vi "1SDI_FPGA_v00.vi"() -> ()   [LabVIEW 2011]
doc: "Controls 6 phase locks based on the interference of two beams at a beam-splitter."
uses:
  Strict Type Defs/Error Signals 1SDI.ctl
  Strict Type Defs/1SDI Lock Point.ctl
  Strict Type Defs/1SDI Output.ctl
  Strict Type Defs/Control 1SDI Input.ctl
  Strict Type Defs/PII individual.ctl
  Strict Type Defs/Error Scale 1SDI.ctl
  Strict Type Defs/Lock Thresh 1SDI.ctl
  Strict Type Defs/Theta graph.ctl
  Strict Type Defs/Safety First.ctl
  Strict Type Defs/Scope.ctl
  Strict Type Defs/1SDI Max.ctl
  Strict Type Defs/1SDI Min.ctl
  <vilib>/rvi/interface/RandomDataEmulation/nirviRandomDataFPGAFIFO.vi
  <vilib>/rvi/interface/RandomDataEmulation/niFpgaRandomDataHandleErrors.vi
  <vilib>/rvi/DataTransferAndStorage/Container/XNode/niFpgaContainer.xnode
  <vilib>/rvi/interface/RandomDataEmulation/nirviRandomDataFpgaReadWriteTemplate.vi
panel:
  out "Min":T1
  out "Max":T2
  in  "Graph Delay(uSec)":u32 caption="Count(uSec)"
  out "HD Errors xp":T3
  in  "Scope":T4={"Trigger Direction"=enum."plus-minus", "Delay"=0, "Aquisition Rate (Ticks)"=40, "Offset"=0, "Channel"=0, "Channel Selector"={"Channel 1"=0, "Channel 2"=4, "Channel 3"=8, "Channel 4"=8}} {"Channel Selector"."Channel 4" items=["Error Signal 1", "Error Signal 2", "Scan Trigger 1", "Scan Trigger 2", "DC Signal 1", "DC Signal 2", "PI Out 1", "PI Out 2"]; "Channel Selector"."Channel 3" items=["Error Signal 1", "Error Signal 2", "Scan Trigger 1", "Scan Trigger 2", "DC Signal 1", "DC Signal 2", "PI Out 1", "PI Out 2"]; "Channel Selector"."Channel 2" items=["Error Signal 1", "Error Signal 2", "Scan Trigger 1", "Scan Trigger 2", "DC Signal 1", "DC Signal 2", "PI Out 1", "PI Out 2"]; "Channel Selector"."Channel 1" items=["Error Signal 1", "Error Signal 2", "Scan Trigger 1", "Scan Trigger 2", "DC Signal 1", "DC Signal 2", "PI Out 1", "PI Out 2"]}
  in  "quit Control Loop":bool
  in  "Control":T5={"PII In 1"={"Lock"=FALSE, "Hold"=FALSE, "P Gain"=0, "P BS"=-5, "I Gain"=0, "I BS"=-10, "I2 G"=0, "I2 BS"=-26, "Scan Amp"=0, "Scan Off"=0, "Scan FS"=0, "SFS BS"=0, "I Max value"=10000, "I2 Max value"=10000, "Scope.Offset"=0, "Trigger Direction"=enum."either", "Scan-PII thresh"=0}, "PII In 2"={"Lock"=FALSE, "Hold"=FALSE, "P Gain"=0, "P BS"=-10, "I Gain"=0, "I BS"=-10, "I2 G"=0, "I2 BS"=-26, "Scan Amp"=0, "Scan Off"=0, "Scan FS"=0, "SFS BS"=0, "I Max value"=10000, "I2 Max value"=10000, "Scope.Offset"=0, "Trigger Direction"=enum."either", "Scan-PII thresh"=0}, "PII In 3"={"Lock"=FALSE, "Hold"=FALSE, "P Gain"=0, "P BS"=-10, "I Gain"=0, "I BS"=-10, "I2 G"=0, "I2 BS"=-26, "Scan Amp"=0, "Scan Off"=0, "Scan FS"=0, "SFS BS"=0, "I Max value"=10000, "I2 Max value"=10000, "Scope.Offset"=0, "Trigger Direction"=enum."either", "Scan-PII thresh"=0}, "Error scale"={"Pre-Offset"={"Pre-Offset 1"=2, "Pre-Offset 2"=0, "Pre-Offset 3"=0, "Pre-Offset 4"=0, "Pre-Offset 5"=2}, "Post-Offset "={"Offset 1"=0, "Offset 2"=300, "Offset 3"=0, "Offset 4"=0, "Offset 5"=0}, "Gains"={"Gain 1"=0, "Gain 2"=300, "Gain 3"=0, "Gain 4"=0, "Gain 5"=0}, "Bit Shifts"={"Bit Shift 1"=0, "Bit Shift 2"=300, "Bit Shift 3"=0, "Bit Shift 4"=0, "Bit Shift 5"=0}}, "Lock Thresh"={"EPR"=2, "HD A"=0, "HD B"=10}, "Re-Scan Thresh"={"EPR"=2, "HD A"=0, "HD B"=0}, "Theta"={"HD A Sin Theta"=0, "HD A Cos Theta"=0, "HD B Sin Theta"=0, "HD B Cos Theta"=0}, "Safety First"={"lim reset"=FALSE, "no limit"=FALSE, "pos slew rate * dt"=0, "neg slew rate * dt"=-10, "Hold All"=FALSE, "Count(Ticks)"=0}}
  in  "\"I too high?\"":T11
  in  "\"Outputs\"":T12
  out "Outputs":T12={"EPR"=-270, "HD A"=-1710, "HD B"=880}
  in  "\"Trigger\"":T11
  out "Trigger":T11
  out "Cavity Errors":T13={"EPR"=0, "HD A"=1800, "HD B"=0}
  out "Control Loop count":i32=11285327
  out "Scope Full?":bool
  out "Scope loop count":i32=119818
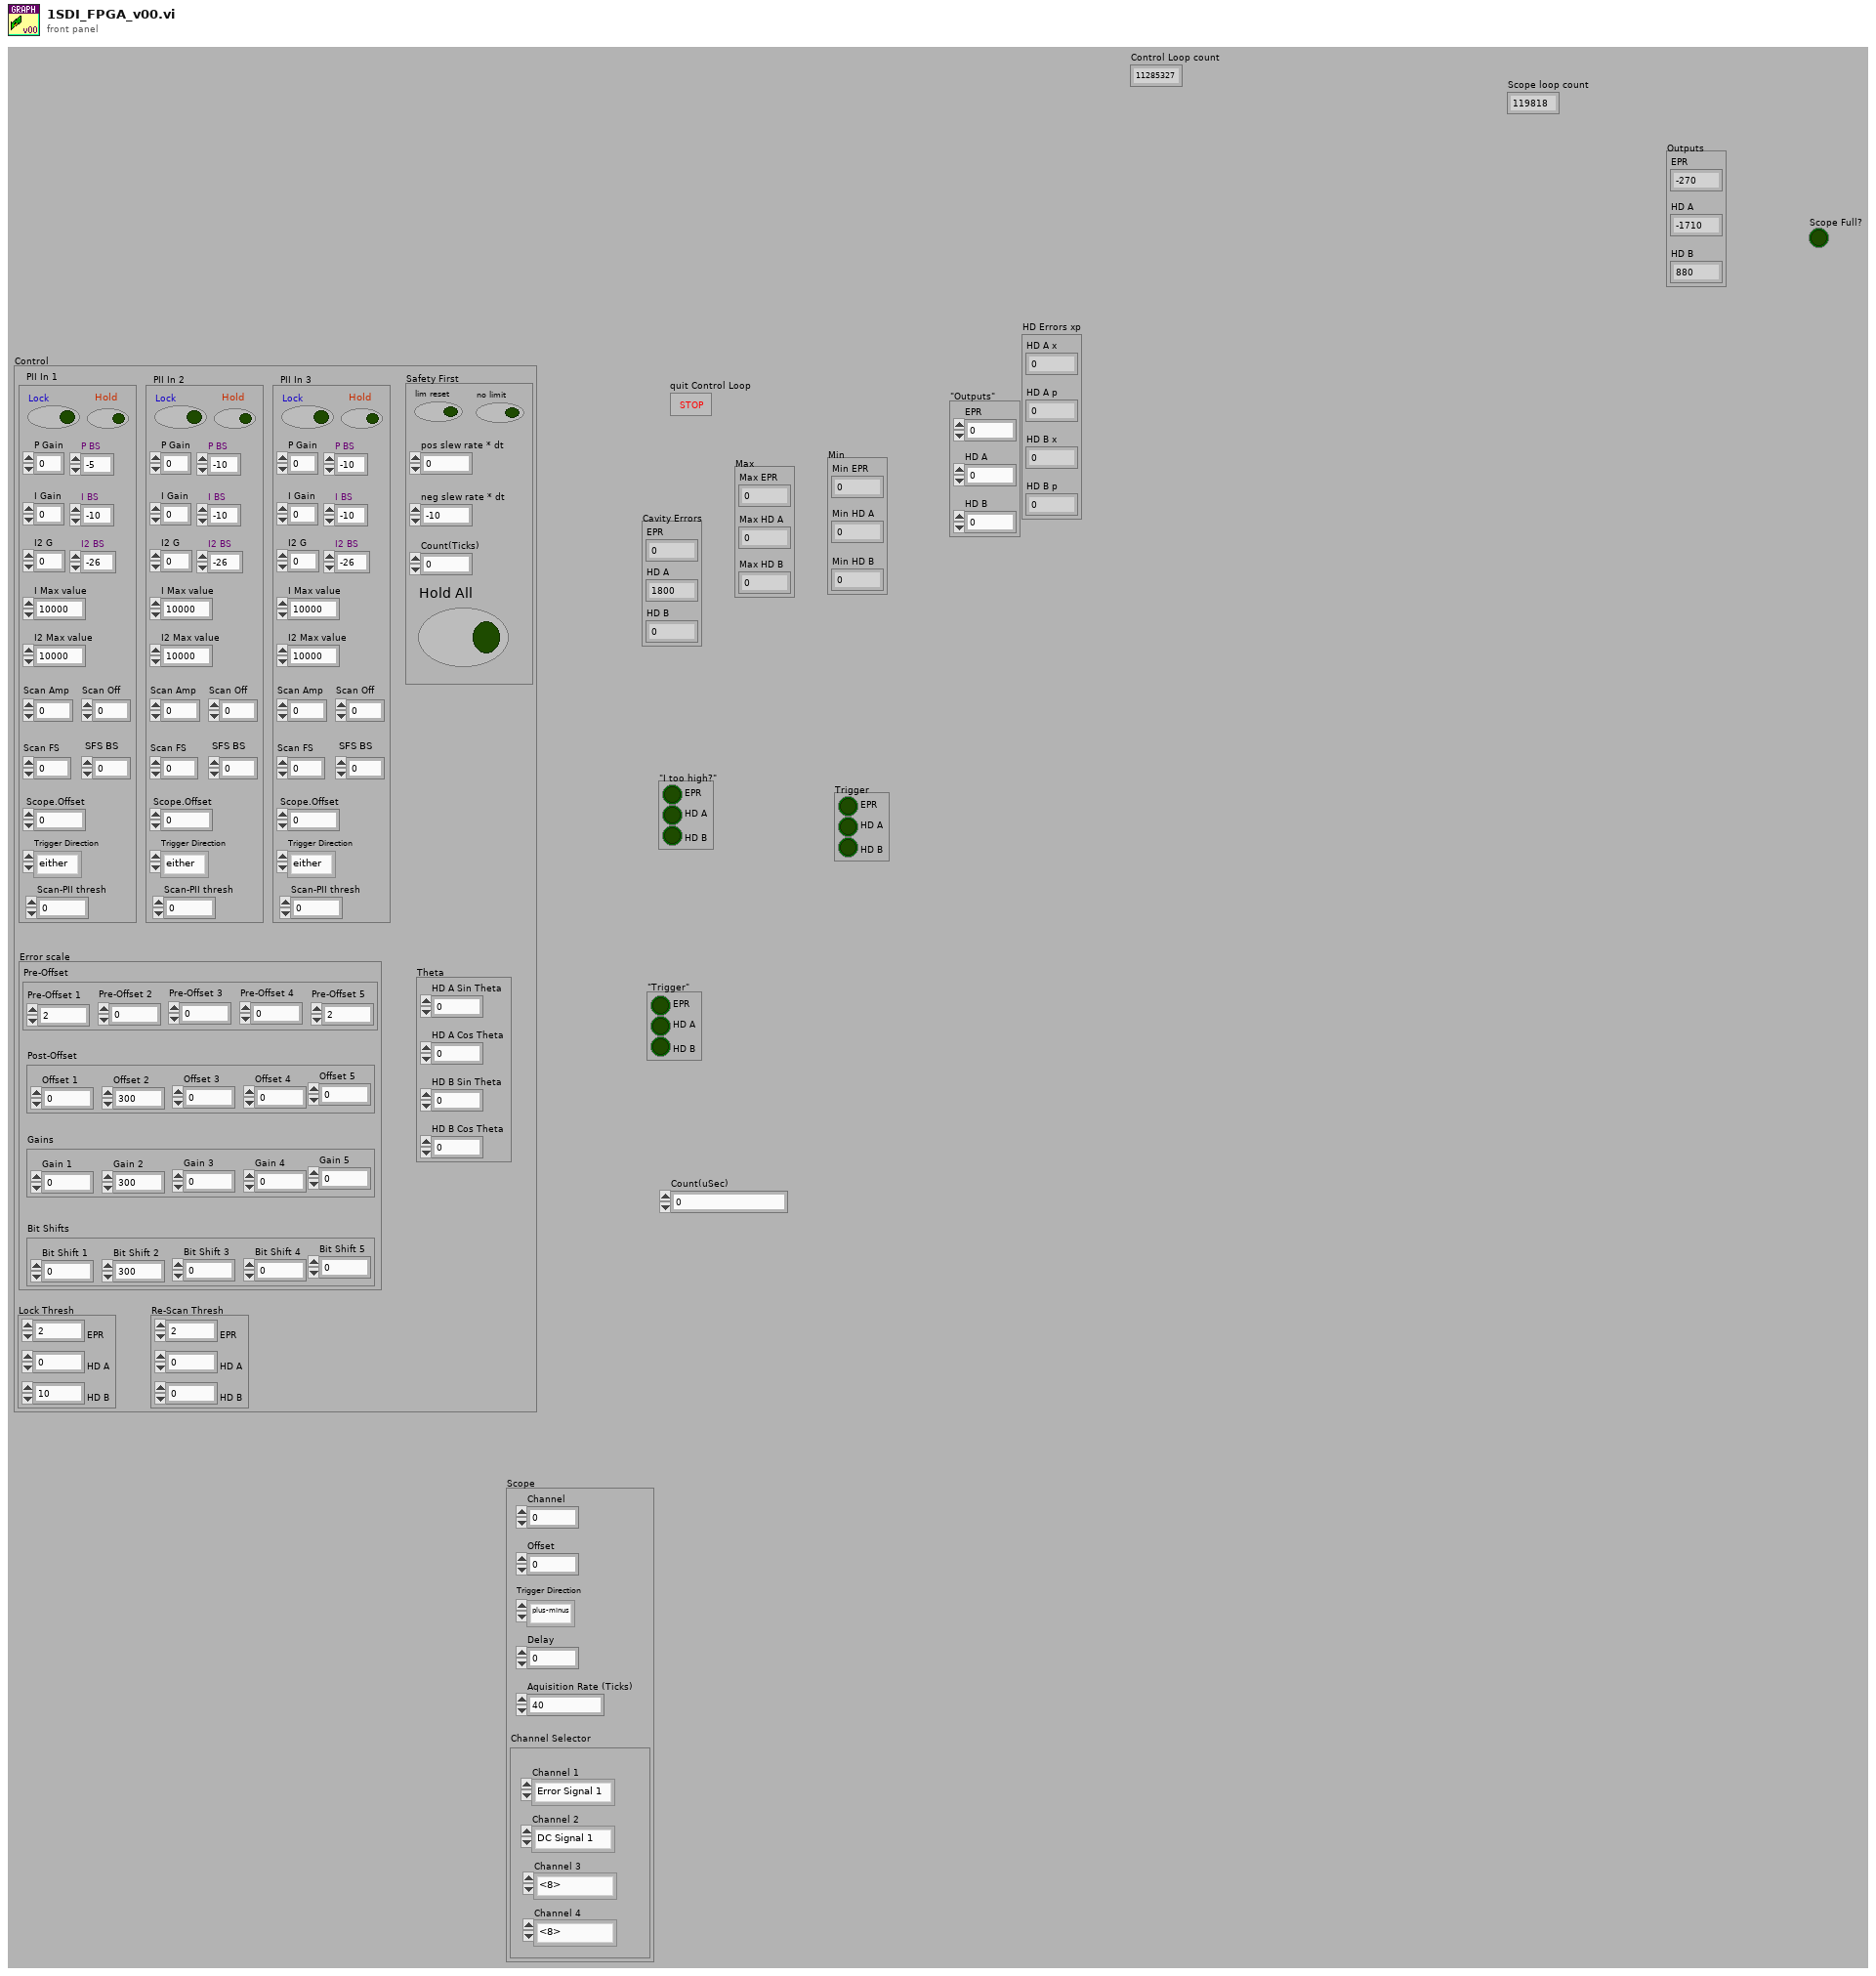
[diagram p1: front panel]
types:
  T1 = typedef "1SDI Min.ctl" = cluster{"Min EPR":i16, "Min HD A":i16, "Min HD B":i16}
  T2 = typedef "1SDI Max.ctl" = cluster{"Max EPR":i16, "Max HD A":i16, "Max HD B":i16}
  T3 = cluster{"HD A x":i16, "HD A p":i16, "HD B x":i16, "HD B p":i16}
  T4 = typedef "Scope.ctl" = cluster{"Trigger Direction":enum8{"either", "minus-plus", "plus-minus"}, "Delay":u32, "Aquisition Rate (Ticks)":u32, "Offset":i16, "Channel":i32, "Channel Selector":cluster{"Channel 1":i32, "Channel 2":i32, "Channel 3":i32, "Channel 4":i32}}
  T5 = typedef "Control 1SDI Input.ctl" = cluster{"PII In 1":T6, "PII In 2":T6, "PII In 3":T6, "Error scale":T7, "Lock Thresh":T8, "Re-Scan Thresh":T8, "Theta":T9, "Safety First":T10}
  T6 = typedef "PII individual.ctl" = cluster{"Lock":bool, "Hold":bool, "P Gain":i32, "P BS":i16, "I Gain":i32, "I BS":i16, "I2 G":i32, "I2 BS":i16, "Scan Amp":i16, "Scan Off":i16, "Scan FS":u16, "SFS BS":i16, "I Max value":i32, "I2 Max value":i32, "Scope.Offset":i16, "Trigger Direction":enum8{"either", "minus-plus", "plus-minus"}, "Scan-PII thresh":i16}
  T7 = typedef "Error Scale 1SDI.ctl" = cluster{"Pre-Offset":cluster{"Pre-Offset 1":i16, "Pre-Offset 2":i16, "Pre-Offset 3":i16, "Pre-Offset 4":i16, "Pre-Offset 5":i16}, "Post-Offset ":cluster{"Offset 1":i16, "Offset 2":i16, "Offset 3":i16, "Offset 4":i16, "Offset 5":i16}, "Gains":cluster{"Gain 1":i16, "Gain 2":i16, "Gain 3":i16, "Gain 4":i16, "Gain 5":i16}, "Bit Shifts":cluster{"Bit Shift 1":i16, "Bit Shift 2":i16, "Bit Shift 3":i16, "Bit Shift 4":i16, "Bit Shift 5":i16}}
  T8 = typedef "Lock Thresh 1SDI.ctl" = cluster{"EPR":i16, "HD A":i16, "HD B":i16}
  T9 = typedef "Theta graph.ctl" = cluster{"HD A Sin Theta":i32, "HD A Cos Theta":i32, "HD B Sin Theta":i32, "HD B Cos Theta":i32}
  T10 = typedef "Safety First.ctl" = cluster{"lim reset":bool, "no limit":bool, "pos slew rate * dt":i16, "neg slew rate * dt":i16, "Hold All":bool, "Count(Ticks)":u32}
  T11 = typedef "1SDI Lock Point.ctl" = cluster{"EPR":bool, "HD A":bool, "HD B":bool}
  T12 = typedef "1SDI Output.ctl" = cluster{"EPR":i16, "HD A":i16, "HD B":i16}
  T13 = typedef "Error Signals 1SDI.ctl" = cluster{"EPR":i16, "HD A":i16, "HD B":i16}
  T14 = typedef "Signals 1SDI.ctl" = cluster{"PII In 1":T6, "PII In 2":T6, "PII In 3":T6, "Lock Thresh":T8, "Re-Scan Thresh":T8, "Safety First":T10, "Graph Errors":T13}
  T15 = typedef "1SDI Control Cluster.ctl" = cluster{"Control EPR":T6, "Control HD A":T6, "Control HD B":T6, "Max":T2, "Min":T1, "Lock Threshold":T8, "Re-Scan Threshold":T8, "Lock Point?":T11, "Re-scan?":T11, "Lock pressed? (-1)":T11, "Cavity Errors":T13, "State (-1)":T16, "Safety First":T10}
  T16 = typedef "1SDI State.ctl" = cluster{"EPR":enum16{"Safe", "Hold", "Scan", "Lock"}, "HD A":enum16{"Safe", "Hold", "Scan", "Lock"}, "HD B":enum16{"Safe", "Hold", "Scan", "Lock"}}
  T17 = typedef "1SDI PII Scan State.ctl" = cluster{"Control EPR":T6, "Control HD A":T6, "Control HD B":T6, "Error Signals":T13, "State":T16}
  T18 = typedef "1SDI MaxMin.ctl" = cluster{"State":T16, "Reset MaxMin?":T19, "Max":T2, "Min":T1, "Lock pressed?":T11, "Safety First":T10}
  T19 = typedef "1SDI Reset MaxMin.ctl" = cluster{"EPR":bool, "HD A":bool, "HD B":bool}
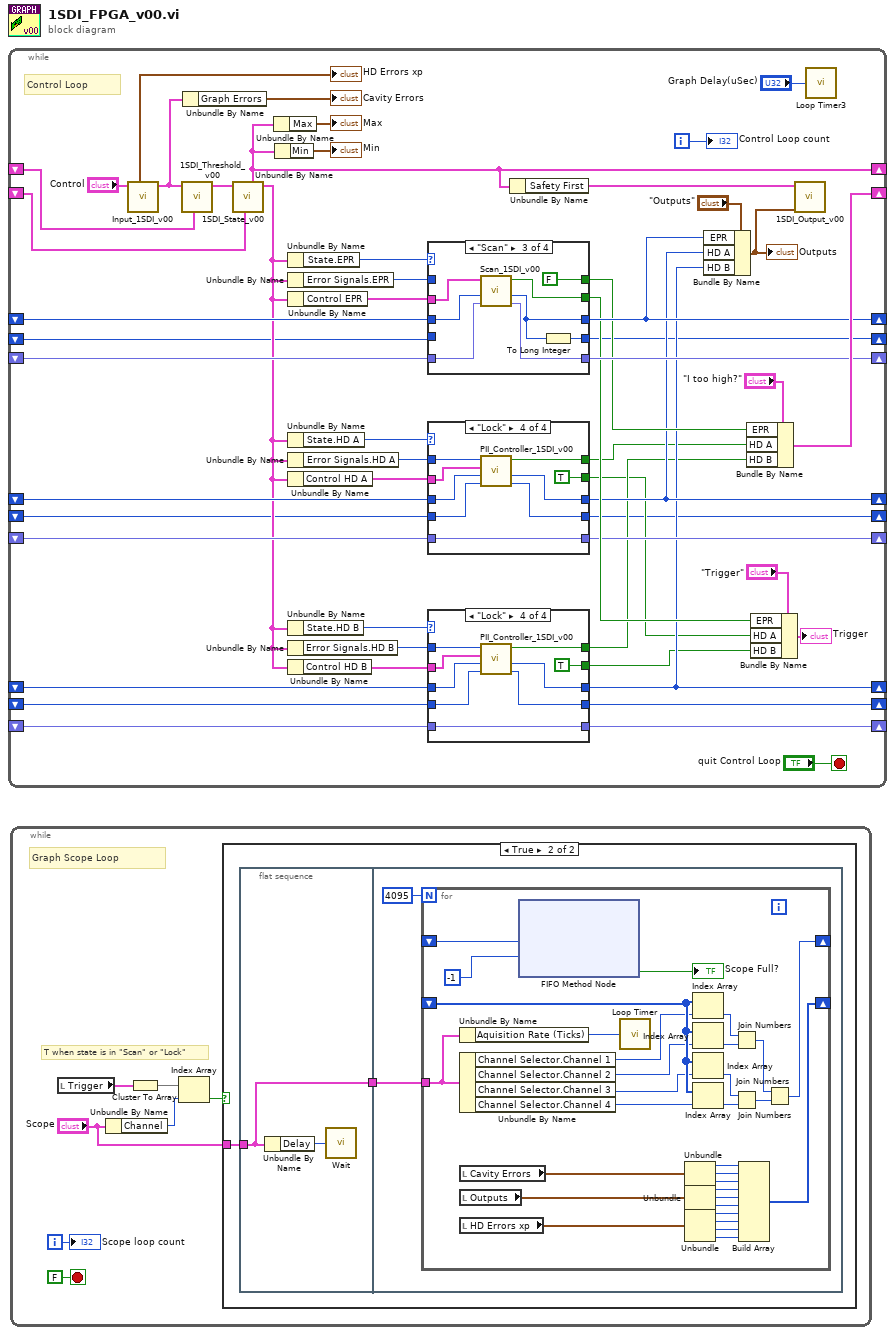
[diagram p0: block diagram]
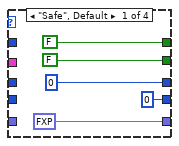
[diagram p3: hidden frame]
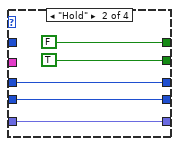
[diagram p4: hidden frame]
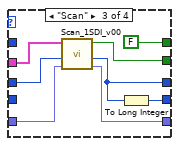
[diagram p5: hidden frame]
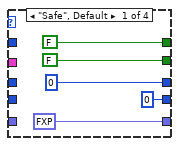
[diagram p6: hidden frame]
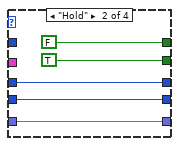
[diagram p7: hidden frame]
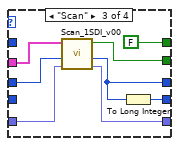
[diagram p8: hidden frame]
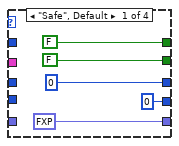
[diagram p9: hidden frame]
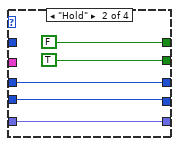
[diagram p10: hidden frame]
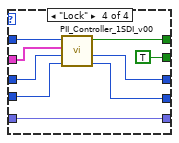
[diagram p11: hidden frame]
diagram:
  n1 = while {
    shift-right: [w53] -> _
    shift-left: _ -> [w48]
    shift-right: [w19] -> _
    shift-left: _ -> [w47]
    shift-right: [w41] -> _
    shift-left: _ -> [w46]
    shift-right: [w45] -> _
    shift-left: _ -> [w44]
    shift-right: [w30] -> _
    shift-left: _ -> [w36]
    shift-right: [w35] -> _
    shift-left: _ -> [w34]
    shift-right: [w2] -> _
    shift-left: _ -> [w1]
    shift-right: [w29] -> _
    shift-left: _ -> [w31]
    shift-right: [w32] -> _
    shift-left: _ -> [w33]
    shift-right: [w6] -> _
    shift-left: _ -> [w5]
    shift-right: [w4] -> _
    shift-left: _ -> [w3]
    i -> [w49]
    stop <- "quit Control Loop" stop-if-true
    # "Control Loop"
    n2 = call "Input_1SDI_v00.vi"("Control"="Control") -> ("Signals"=w24:T14, "HD Errors xp"=→"HD Errors xp":T3)  [unwired: 9 in]
    n3 = call "1SDI_Threshold_v00.vi"("MaxMin"=w47, "Signals"=w24) -> ("Control Graph Cluster"=w21:T15)  [unwired: 9 in]
    n4 = Unbundle By Name(w24) -> ("Graph Errors"=→"Cavity Errors":T13)
    n5 = call "1SDI_State_v00.vi"("\"I too high?\""=w48, "Control Cavity Cluster"=w21) -> ("PII Scan State Errors"=w8:T17, "MaxMin"=w19:T18)  [unwired: 8 in]
    n6 = Unbundle By Name(w19) -> ("Max"=→"Max":T2)
    n7 = Unbundle By Name(w19) -> ("Min"=→"Min":T1)
    n8 = Unbundle By Name(w8) -> ("State.EPR"=w15:enum16{"Safe", "Hold", "Scan", "Lock"})
    n9 = Unbundle By Name(w8) -> ("Error Signals.EPR"=w16:i16)
    n10 = Unbundle By Name(w8) -> ("Control EPR"=w17:T6)
    n11 = Unbundle By Name(w8) -> ("State.HD A"=w14:enum16{"Safe", "Hold", "Scan", "Lock"})
    n12 = Unbundle By Name(w8) -> ("Error Signals.HD A"=w13:i16)
    n13 = Unbundle By Name(w8) -> ("Control HD A"=w12:T6)
    n14 = Unbundle By Name(w8) -> ("State.HD B"=w9:enum16{"Safe", "Hold", "Scan", "Lock"})
    n15 = Unbundle By Name(w8) -> ("Error Signals.HD B"=w11:i16)
    n16 = Unbundle By Name(w8) -> ("Control HD B"=w10:T6)
    n17 = case shown="\"Scan\"" w15 {
      tunnel: w16 -> [_ _ _ w135]
      tunnel: [FALSE ("I too high? (F=No)") FALSE ("I too high? (F=No)") FALSE ("I too high? (F=No)") w134] -> w40
      tunnel: w17 -> [_ _ w125 w133]
      tunnel: [i16 0 ("PII out") w117 w119 w130] -> w41
      tunnel: w46 -> [_ w117 w122 w131]
      tunnel: w3 -> [_ w114 _ w127]
      tunnel: [fxp<+,33,17> 0.0 ("Scan") w116 w124 w129] -> w45
      tunnel: w44 -> [_ w116 w123 w129]
      tunnel: [FALSE ("Zero Crossing") TRUE ("Zero Crossing") w121 TRUE ("Zero Crossing")] -> w39
      tunnel: [0 ("I Cavity") w114 w120 w128] -> w4
      frame "Safe", Default {
      }
      frame "Hold" {
      }
      frame "Scan" {
        n18 = call "Scan_1SDI_v00.vi"("Scan (-1)"=w123, "Scan out (-1)"=w122, "Control Cavity"=w125) -> ("Scan"=w124:fxp<+,33,17>, "Scan out"=w119:i16, "Zero Crossing"=w121:bool)  [unwired: 6 in]
        n19 = To Long Integer(number=w119) -> (32bit integer=w120:i32)
      }
      frame "Lock" {
        n20 = call "PII_Controller_1SDI_v00.vi"("Integrator (-1)"=w127, "PII out (-1)"=w131, "Control Cavity"=w133, "OPO A Error"=w135) -> ("I Cavity"=w128:i32, "PII out"=w130:i16, "I too high?"=w134:bool)  [unwired: 5 in]
      }
    }
    n21 = case shown="\"Lock\"" w14 {
      tunnel: w13 -> [_ _ _ w108]
      tunnel: [FALSE ("I too high? (F=No)") FALSE ("I too high? (F=No)") FALSE ("I too high? (F=No)") w107] -> w28
      tunnel: w12 -> [_ _ w98 w105]
      tunnel: [i16 0 ("PII out") w90 w92 w102] -> w30
      tunnel: w36 -> [_ w90 w95 w103]
      tunnel: w5 -> [_ w87 _ w106]
      tunnel: [fxp<+,33,17> 0.0 ("Scan") w89 w97 w101] -> w35
      tunnel: w34 -> [_ w89 w96 w101]
      tunnel: [FALSE ("Zero Crossing") TRUE ("Zero Crossing") w94 TRUE ("Zero Crossing")] -> w26
      tunnel: [0 ("I Cavity") w87 w93 w100] -> w6
      frame "Safe", Default {
      }
      frame "Hold" {
      }
      frame "Scan" {
        n22 = call "Scan_1SDI_v00.vi"("Scan (-1)"=w96, "Scan out (-1)"=w95, "Control Cavity"=w98) -> ("Scan"=w97:fxp<+,33,17>, "Scan out"=w92:i16, "Zero Crossing"=w94:bool)  [unwired: 6 in]
        n23 = To Long Integer(number=w92) -> (32bit integer=w93:i32)
      }
      frame "Lock" {
        n24 = call "PII_Controller_1SDI_v00.vi"("Integrator (-1)"=w106, "PII out (-1)"=w103, "Control Cavity"=w105, "OPO A Error"=w108) -> ("I Cavity"=w100:i32, "PII out"=w102:i16, "I too high?"=w107:bool)  [unwired: 5 in]
      }
    }
    n25 = case shown="\"Lock\"" w9 {
      tunnel: w11 -> [_ _ _ w81]
      tunnel: [FALSE ("I too high? (F=No)") FALSE ("I too high? (F=No)") FALSE ("I too high? (F=No)") w80] -> w27
      tunnel: w10 -> [_ _ w71 w79]
      tunnel: [i16 0 ("PII out") w63 w66 w76] -> w29
      tunnel: w31 -> [_ w63 w68 w77]
      tunnel: [fxp<+,33,17> 0.0 ("Scan") w62 w70 w75] -> w32
      tunnel: w33 -> [_ w62 w69 w75]
      tunnel: [FALSE ("Zero Crossing") TRUE ("Zero Crossing") w67 TRUE ("Zero Crossing")] -> w25
      tunnel: [0 ("I Cavity") w60 w65 w74] -> w2
      tunnel: w1 -> [_ w60 _ w73]
      frame "Safe", Default {
      }
      frame "Hold" {
      }
      frame "Scan" {
        n26 = call "Scan_1SDI_v00.vi"("Scan (-1)"=w69, "Scan out (-1)"=w68, "Control Cavity"=w71) -> ("Scan"=w70:fxp<+,33,17>, "Scan out"=w66:i16, "Zero Crossing"=w67:bool)  [unwired: 6 in]
        n27 = To Long Integer(number=w66) -> (32bit integer=w65:i32)
      }
      frame "Lock" {
        n28 = call "PII_Controller_1SDI_v00.vi"("Integrator (-1)"=w73, "PII out (-1)"=w77, "Control Cavity"=w79, "OPO A Error"=w81) -> ("I Cavity"=w74:i32, "PII out"=w76:i16, "I too high?"=w80:bool)  [unwired: 5 in]
      }
    }
    n29 = Unbundle By Name(w19) -> ("Safety First"=w43:T10)
    n30 = Bundle By Name(cluster="\"Outputs\"", "EPR"=w41, "HD A"=w30, "HD B"=w29) -> (w42:T12)
    "Outputs" <- w42
    n31 = Bundle By Name(cluster="\"I too high?\"", "EPR"=w40, "HD A"=w28, "HD B"=w27) -> (w53:T11)
    n32 = Bundle By Name(cluster="\"Trigger\"", "EPR"=w39, "HD A"=w26, "HD B"=w25) -> (→"Trigger":T11)
    n33 = call "1SDI_Output_v00.vi"("Outputs"=w42, "Safety First"=w43) -> ()  [unwired: 10 in]
    n34 = call "Loop Timer3"("Count(uSec)"="Graph Delay(uSec)") -> ()  [unwired: 1 out]
    "Control Loop count" <- w49
  }
  n35 = while {
    i -> [w139]
    stop <- FALSE ("stop") stop-if-true
    # "Graph Scope Loop"
    # "T when state is in \"Scan\" or \"Lock\""
    n36 = local read "Trigger"() -> (w137:T11)
    n37 = Unbundle By Name("Scope") -> ("Channel"=w140:i32)
    n38 = Cluster To Array(cluster=w137) -> (array=w141:bool[])
    n39 = Index Array(array=w141, index=w140) -> (element=w138:bool)
    n40 = case shown="True" w138 {
      tunnel: "Scope" -> [_ w144]
      frame False {
      }
      frame True {
        n41 = flat-sequence {
          tunnel: w144 -> [w145]
          tunnel: [w145] -> w143
          tunnel: w143 -> [w147]
          frame #0 {
            n42 = Unbundle By Name(w145) -> ("Delay"=w146:u32)
            n43 = call "Wait"("Count(Ticks)"=w146) -> ()  [unwired: 1 out]
          }
          frame #1 {
            n44 = for {
              N: 4095 -> [_]
              tunnel: w147 -> [w178]
              shift-right: [w170] -> _
              shift-left: _ -> [w169]
              shift-right: [w165] -> _
              shift-left: _ -> [w164]
              n45 = Unbundle By Name(w178) -> ("Aquisition Rate (Ticks)"=w179:u32)
              n46 = Unbundle By Name(w178) -> ("Channel Selector.Channel 1"=w166:i32, "Channel Selector.Channel 2"=w167:i32, "Channel Selector.Channel 3"=w161:i32, "Channel Selector.Channel 4"=w168:i32)
              n47 = local read "Cavity Errors"() -> (w177:T13)
              n48 = local read "Outputs"() -> (w176:T12)
              n49 = local read "HD Errors xp"() -> (w159:T3)
              n50 = xnode ("FIFO Method Node")("Element"=w164, "Timeout"=-1) -> ("Timed Out?"=→"Scope Full?":bool)  [unwired: 1 in, 1 out]
              n51 = call "Loop Timer"("Count(uSec)"=w179) -> ()  [unwired: 1 out]
              n52 = Unbundle(w177) -> ("EPR"=w149:i16, "HD A"=w150:i16, "HD B"=w151:i16)
              n53 = Unbundle(w176) -> ("EPR"=w152:i16, "HD A"=w153:i16, "HD B"=w154:i16)
              n54 = Unbundle(w159) -> ("HD A x"=w158:i16, "HD A p"=w157:i16, "HD B x"=w156:i16, "HD B p"=w155:i16)
              n55 = Index Array(array=w169, index=w166) -> (element=w172:i16)
              n56 = Index Array(array=w169, index=w167) -> (element=w171:i16)
              n57 = Index Array(array=w169, index=w161) -> (element=w160:i16)
              n58 = Index Array(array=w169, index=w168) -> (element=w173:i16)
              n59 = Join Numbers(hi=w172, lo=w171) -> ((hi.lo)=w175:u32)
              n60 = Join Numbers(hi=w160, lo=w173) -> ((hi.lo)=w174:u32)
              n61 = Build Array(w149, w150, w151, w152, w153, w154, w158, w157, w156, w155) -> (w170:i16[])
              n62 = Join Numbers(hi=w175, lo=w174) -> ((hi.lo)=w165:u64)
            }
          }
        }
      }
    }
    "Scope loop count" <- w139
  }
